vi "Cmd Get String Parameter Value (CR).vi"(6 "error in (no error)":errorcluster, 7 "type":string, 8 "parameter index":variant, 9 "command-recordset reference":T1) -> (0 "error out":errorcluster, 1 "value":string, 3 "command-recordset reference out":T1)   [LabVIEW 2020, in "NI_Database_API.lvlib"]
doc: "Retrieves the value of the parameter specified by the <B>parameter index</B> input in the command or command-recordset. The <B>parameter index</B> can be either the zero-indexed position of the parameter in the command or the name of the parameter. Wire data to the <B>type</B> input to determine the polymorphic instance to use or manually select the instance."
uses:
  <vilib>/addons/database/NI_Database_API.lvlib
  <vilib>/addons/database/Command-Recordset.llb/Cmd-Rec Object Reference.ctl
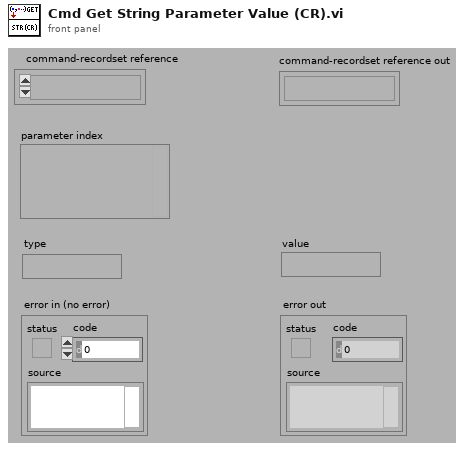
[diagram p1: front panel]
types:
  T1 = typedef "NI_Database_API.lvlib/Cmd-Rec Object Reference.ctl" = refnum<k1>
  T2 = typedef "NI_Database_API.lvlib/Cmd-Rec Data Members.ctl" = cluster{"recordset reference":T3, "command reference":T4}
  T3 = typedef "NI_Database_API.lvlib/Rec ObjectReference.ctl" = refnum<k1>
  T4 = typedef "NI_Database_API.lvlib/Cmd ObjectReference.ctl" = refnum<k1>
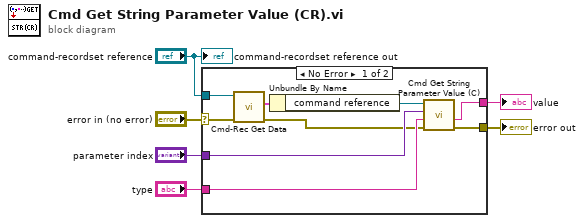
[diagram p0: block diagram]
diagram:
  n1 = case shown="No Error" "error in (no error)" {
    selector: "error in (no error)" -> [w7 w16]
    tunnel: "parameter index" -> [w15 _]
    tunnel: "type" -> [w14 _]
    tunnel: [w13 _] -> w4
    tunnel: [w12 w16] -> w3
    tunnel: "command-recordset reference" -> [w8 _]
    frame No Error {
      n2 = call <vilib>:"Cmd-Rec Get Data.vi"("error in (no error)"=w7, "command-recordset reference"=w8) -> ("error out"=w9:errorcluster, "data"=w10:T2)  [unwired: 2 in, 2 out]
      n3 = Unbundle By Name(w10) -> ("command reference"=w11:T4)
      n4 = call <vilib>:"Cmd Get String Parameter Value (C).vi"("error in (no error)"=w9, "type"=w14, "parameter index"=w15, "command reference"=w11) -> ("error out"=w12:errorcluster, "value"=w13:string)  [unwired: 3 in, 1 out]
    }
    frame Error {
    }
  }
  "error out" <- w3
  "value" <- w4
  "command-recordset reference out" <- "command-recordset reference"
